vi "BlockAngle.vi"(7 "target":dbl[](array[numeric]), 8 "error in (no error)":errorcluster, 9 "Game ref":refnum<class "Game.lvclass">, 10 "Robot in":refnum<class "Robot.lvclass">, 11 "DefendAreaTactic in":refnum<class "DefendAreaTactic.lvclass">) -> (0 "error out":errorcluster, 2 "Robot out":refnum<class "Robot.lvclass">, 3 "DefendAreaTactic out":refnum<class "DefendAreaTactic.lvclass">)   [LabVIEW 2024, in "DefendAreaTactic.lvclass"]
uses:
  DefendAreaTactic.lvclass
  Game_class/Game.lvclass
  Robot_class/Robot.lvclass
  C:/Users/as119/OneDrive/Documentos/roboIME/SSL_AI/Object_class/Object.lvclass
  WallPositions.ctl
  Game_class/Game.lvclass/Game.ctl
  Team_class/Team.lvclass/Team.ctl
  Robot_class/Robot.lvclass/Robot.ctl
  Object_class/Object.lvclass/Object.ctl
  Field_class/Field.lvclass/Field.ctl
  Robot_class/Read id.vi
  Object_class/Read position(x,y).vi
  Object_class/Read y.vi
  Robot_class/Read v_norm.vi
  Robot_class/Read orientation.vi
  Game_class/Read FieldRef.vi
  Game_class/Read DefensiveTeam.vi
  Game_class/Read NewParameters.vi
  Team_class/Read RobotRef.vi
  Robot_class/Read dest_x.vi
  Robot_class/Read dest_y.vi
  Field_class/Read ourGoalPosition.vi
  Robot_class/Write dest_orientation.vi
  Robot_class/Write dest_x.vi
  Robot_class/Write dest_y.vi
  Robot_class/Write kick_x.vi
  Robot_class/Write kick_z.vi
  Ally_class/Ally.lvclass
  C:/Users/as119/OneDrive/Documentos/roboIME/SSL_AI/Team_class/Team.lvclass
  Field_class/Field.lvclass
  <vilib>/Analysis/NI_AALPro.lvlib
  Utilities_class/Utilities.lvclass
  <vilib>/Analysis/coordinate.llb/2D Cartesian Coordinate Rotation (Scalar).vi
  Ball_class/Ball.lvclass
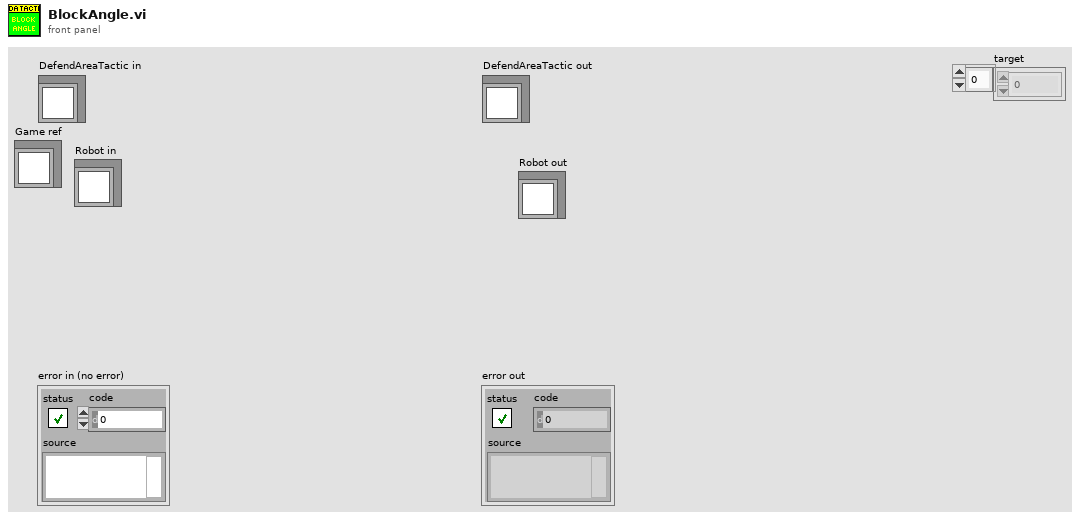
[diagram p1: front panel]
types:
  T1 = typedef "WallPositions.ctl" = enum16{"LeftWall", "LeftCorner", "FrontWall", "RightCorner", "RightWall"}
  T2 = typedef "NewParameters.ctl" = cluster{"PenaltyDistance":dbl, "DistanceAttackerToBackBall":dbl, "Division":enum16{"Div B", "Div A"}, "DistanceToAvoidyEnemyRobot":dbl, "BallPlacementDistance":dbl, "DisatanceBehindBallToStealBall":dbl, "MaxDistanceToPositionKickoff":dbl, "BlockEnemyTarget":bool, "MaxStopVAng":dbl, "DistanceMarkerToEnemy":dbl, "IgnoreDribblerContact":bool, "DistanceToBeginEnemyPosession":dbl, "GoToBallWhenEnemyNotMoving":bool, "EnemyDistanceToReduceVelocity":dbl, "TurnOnEnemyDistanceToReduceVelocity":bool, "EnemyDistanceToShootOutBall":dbl, "DefenseKickBall":bool, "MoreKickToGoal? (0-0.3)":dbl, "ChipKickInEnemyField":bool, "ShootOutRobotId":dbl, "FieldLenghtDenominatorInShootOut":dbl, "AdjustPositionInBallPlacement":bool, "PowerGodPass":dbl, "VelocityAbortEnemyPos":dbl, "MaxDistToBeginPass":dbl, "MinDistToBeginPass":dbl, "VelocityInDirects":dbl, "BadDribblerIDs":i32[], "NewKickToDistanceAroundBall":dbl, "PowerAvoidColisionMarker":dbl, "DistanceToAvoidColisionMarker":dbl, "AvoidBallKick":dbl, "DistanceTryKick":dbl, "SuicideKickDIstance":dbl, "AdjustFirstKickDistance":dbl, "AvoidAimLessKick":dbl, "DistanceToAvoidyEnemyShootRobot ":dbl, "NumberOfMarkers":dbl, "PotField":bool, "PIDLateral":bool, "MinDistanceFirstKickX":dbl, "MinDistanceFirstKickY":dbl, "FractionOfDistToTouchGround\nAfterChipKick":dbl, "FractionOfKickxWhen\nComposedWithKickz":dbl, "Style":T3, "MoveInTurnState":bool, "DistFromEnemyToConsider\nMoveInTurnState":dbl, "CascadePID":bool, "TurnAroundParameters":cluster{"Radius":dbl, "Multiplier":dbl, "ChordAngle":dbl}, "SafeDriveVel":dbl, "DistanceToGoToBackBall":dbl, "minDistanceToNotFinish\nEnemyPossession":dbl, "OneTouchShot":cluster{"angleFactor":dbl, "maxAngle":dbl, "Attack":bool, "Defense":bool}, "OpenAngleToGoal":cluster{"minAngle":dbl, "maxAngle":dbl, "minEvaluation":dbl}, "ShotInterception":cluster{"shotSpeed":dbl, "minEnemySpeed":dbl, "maxEnemySpeed":dbl, "minEvaluation":dbl}, "AllyTeamArray":T4[], "maxDefendersNumber":i32, "Zone":cluster{"GuardPositionArray":dbl[][], "ZoneMidField":dbl[], "CenterForwardWidth":dbl}, "MinEvaluationToShoot":dbl, "PassInterception":cluster{"maxPassSpeed":dbl, "minPassSpeed":dbl, "minEnemySpeed":dbl, "chipPassDistance":dbl, "chipPassEvaluation":dbl, "minEvaluation":dbl, "maxEnemySpeed":dbl}, "PassDistance":cluster{"maxDistance":dbl, "minDistance":dbl}, "receiverSpeed":dbl, "maxBallSpeed":dbl, "slackTime":dbl, "Turning radius":dbl, "Turning v_ang":dbl, "AlignError":cluster{"Distance":dbl, "Orientation":dbl, "V_norm(m/s)":dbl, "V_ang (rad/s)":dbl}, "RobotRadius":dbl, "KickerDistance":dbl, "keeper angle  to cover goalpost":dbl, "a_slide":dbl, "a_roll":dbl, "k_switch":dbl}
  T3 = typedef "Style.ctl" = enum16{"Insanity", "Offensive", "Defensive"}
  T4 = typedef "AllyTeam.ctl" = enum16{"Keeper", "Defender", "Attacker"}
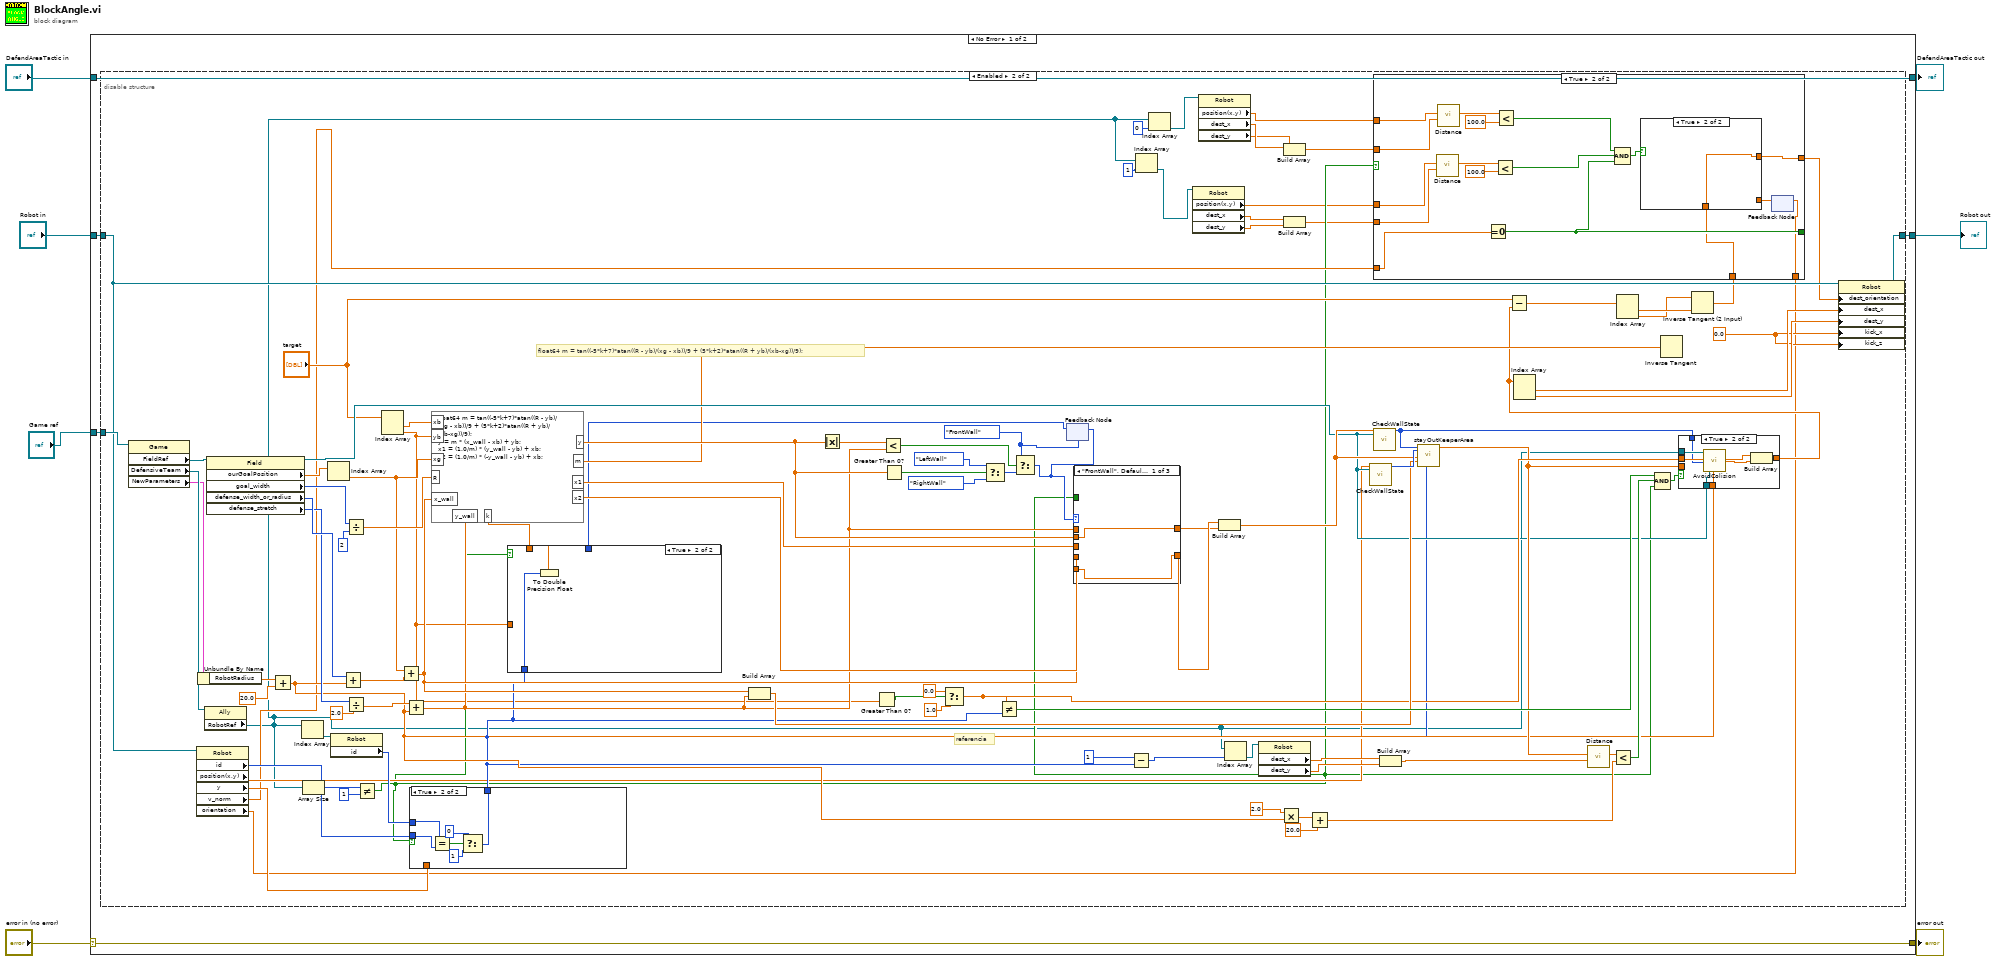
[diagram p0: block diagram]
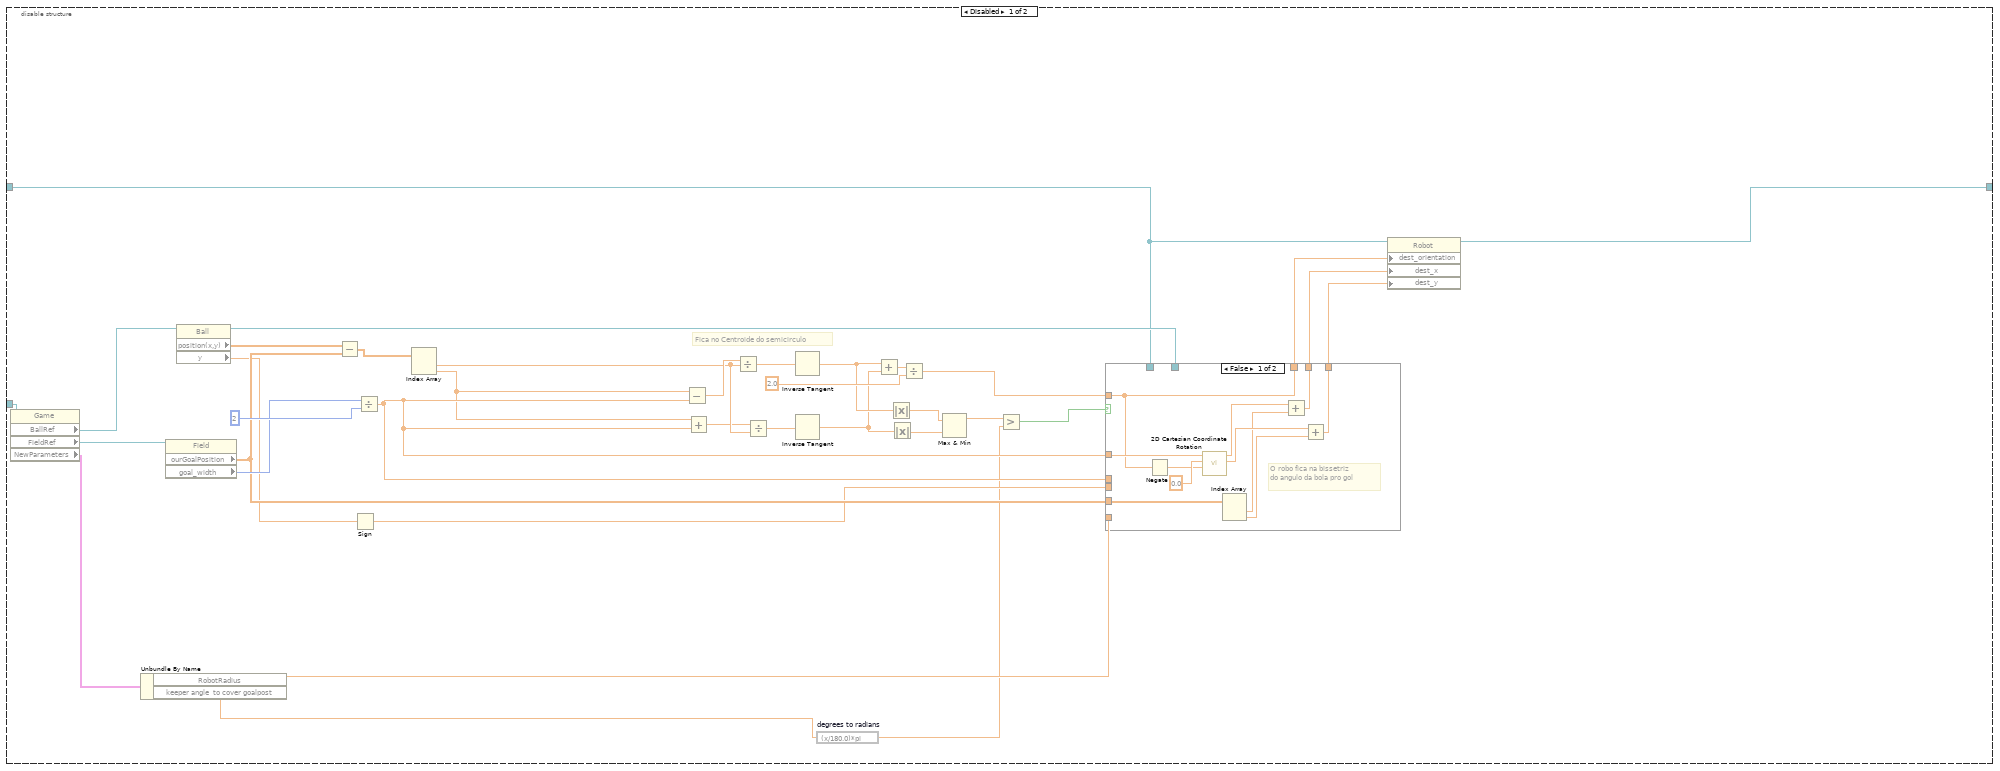
[diagram p2: hidden frame]
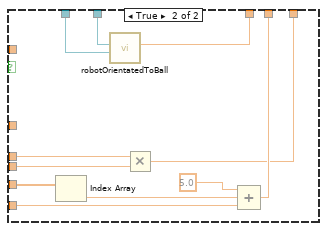
[diagram p3: hidden frame]
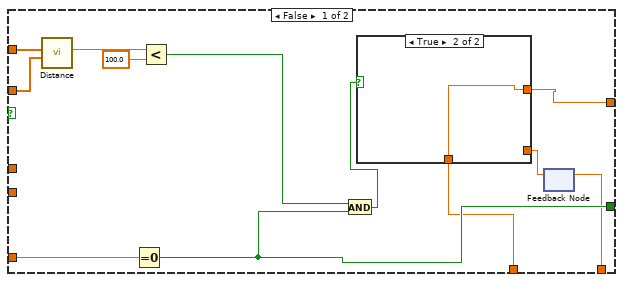
[diagram p4: hidden frame]
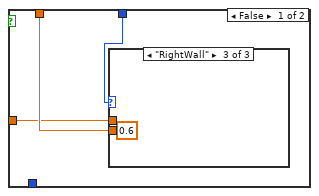
[diagram p7: hidden frame]
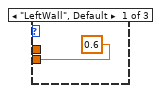
[diagram p8: hidden frame]
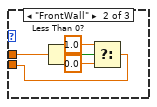
[diagram p9: hidden frame]
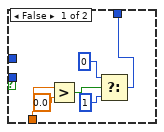
[diagram p10: hidden frame]
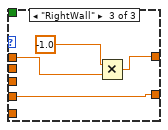
[diagram p13: hidden frame]
diagram:
  n1 = case shown="No Error" "error in (no error)" {
    selector: "error in (no error)" -> [w11 w244]
    tunnel: [w11 w244] -> w6
    tunnel: [w12 w243] -> w4
    tunnel: "DefendAreaTactic in" -> [w12 w243]
    tunnel: "Game ref" -> [w10 _]
    tunnel: "Robot in" -> [w8 w242]
    tunnel: [w9 w242] -> w1
    frame No Error {
      n2 = disable-structure shown="Enabled" {
        disable-tunnel: w10 -> [w23 w167]
        disable-tunnel: [w22 w157] -> w9
        disable-tunnel: w8 -> [w21 w155]
        frame Disabled {
          # "Fica no Centroide do semicirculo"
          n3 = property class="Game"(reference=w23) -> ("BallRef"=w48:refnum<class "Ball.lvclass">, "FieldRef"=w47:refnum<class "Field.lvclass">, "NewParameters"=w29:T2)  [unwired: 1 in, 2 out]
          n4 = Unbundle By Name(w29) -> ("RobotRadius"=w28:dbl, "keeper angle  to cover goalpost"=w13:dbl)
          n5 = property class="Field"(reference=w47) -> ("ourGoalPosition"=w35:dbl[], "goal_width"=w36:i32)  [unwired: 1 in, 2 out]
          n6 = property class="Ball"(reference=w48) -> (reference out=w30:refnum<class "Ball.lvclass">, "position(x,y)"=w46:dbl[], "y"=w25:dbl)  [unwired: 1 in, 1 out]
          n7 = Subtract(x=w46, y=w35) -> (x-y=w44:dbl[])
          n8 = Sign(1:w25) -> (0:w24:dbl)
          n9 = Divide(x=w36, y=2) -> (x/y=w27:dbl)
          n10 = Index Array(array=w44) -> (element #1=w42:dbl, element #2=w26:dbl)  [unwired: 2 in]
          n11 = Subtract(x=w26, y=w27) -> (x-y=w43:dbl)
          n12 = Add(x=w26, y=w27) -> (x+y=w41:dbl)
          n13 = Divide(x=w43, y=w42) -> (x/y=w45:dbl)
          n14 = Divide(x=w41, y=w42) -> (x/y=w40:dbl)
          n15 = Inverse Tangent(1:w45) -> (0:w20:dbl)
          n16 = Inverse Tangent(1:w40) -> (0:w19:dbl)
          n17 = expression code="(x/180.0)*pi" "degrees to radians"(w13) -> (w15:dbl)
          n18 = Add(x=w20, y=w19) -> (x+y=w38:dbl)
          n19 = Absolute Value(x=w20) -> (abs(x)=w18:dbl)
          n20 = Absolute Value(x=w19) -> (abs(x)=w17:dbl)
          n21 = Divide(x=w38, y=2.0) -> (x/y=w32:dbl)
          n22 = Max & Min(x=w18, y=w17) -> (max(x,y)=w16:dbl)  [unwired: 1 out]
          n23 = Greater?(x=w16, y=w15) -> (0:w14:bool)
          n24 = case shown="False" w14 {
            tunnel: w27 -> [w58 _]
            tunnel: w35 -> [w57 w67]
            tunnel: [w51 w64] -> w34
            tunnel: [w50 w61] -> w33
            tunnel: w32 -> [w49 _]
            tunnel: [w49 w69] -> w31
            tunnel: w30 -> [_ w70]
            tunnel: w28 -> [_ w68]
            tunnel: w27 -> [_ w62]
            tunnel: w24 -> [_ w63]
            tunnel: w21 -> [_ w60]
            frame False {
              # "O robo fica na bissetriz \ndo angulo da bola pro gol"
              n25 = Negate(x=w49) -> (-x=w54:dbl)
              n26 = call-poly <vilib>:"2D Cartesian Coordinate Rotation.vi"("theta"=w54, "y"=0.0, "x"=w58) -> ("y out"=w55:dbl, "x out"=w56:dbl)  [unwired: 6 in, 1 out]
              n27 = Index Array(array=w57) -> (element #1=w53:dbl, element #2=w52:dbl)  [unwired: 2 in]
              n28 = Add(x=w56, y=w53) -> (x+y=w51:dbl)
              n29 = Add(x=w55, y=w52) -> (x+y=w50:dbl)
            }
            frame True {
              n30 = Index Array(array=w67) -> (element=w66:dbl)  [unwired: 1 in]
              n31 = call "robotOrientatedToBall.vi"("Robot"=w60, "BallRef"=w70) -> ("Orientation"=w69:dbl)  [unwired: 7 in, 2 out]
              n32 = Multiply(x=w62, y=w63) -> (x*y=w61:dbl)
              n33 = Compound Arithmetic op=ADD(5.0 ("value"), w66, w68) -> (w64:dbl)
            }
          }
          n34 = property class="Robot"(reference=w21, "dest_orientation"=w31, "dest_x"=w34, "dest_y"=w33) -> (reference out=w22:refnum<class "Robot.lvclass">)  [unwired: 1 in, 1 out]
        }
        frame Enabled {
          w89 = 0.0 ("kick_x")
          w94 = WallPositions."FrontWall"
          # "float64 m = tan((-5*k+7)*atan((R - yb)/(xg - xb))/9 + (5*k+2)*atan((R + yb)/(xb-xg))/9);"
          # "referencia"
          n35 = property class="Game"(reference=w167) -> ("FieldRef"=w166:refnum<class "Field.lvclass">, "DefensiveTeam"=w156:refnum<class "Ally.lvclass">, "NewParameters"=w135:T2)  [unwired: 1 in, 2 out]
          n36 = property class="Robot"(reference=w155) -> ("id"=w152:i32, "position(x,y)"=w91:dbl[], "y"=w121:dbl, "v_norm"=w88:dbl, "orientation"=w71:dbl)  [unwired: 1 in, 2 out]
          n37 = Unbundle By Name(w135) -> ("RobotRadius"=w107:dbl)
          n38 = property class="Ally"(reference=w156) -> ("RobotRef"=w85:refnum<class "Robot.lvclass">[])  [unwired: 1 in, 2 out]
          n39 = property class="Field"(reference=w166) -> (reference out=w109:refnum<class "Field.lvclass">, "ourGoalPosition"=w164:dbl[], "goal_width"=w163:i32, "defense_width_or_radius"=w151:i32, "defense_stretch"=w149:i32)  [unwired: 1 in, 1 out]
          n40 = Add(x=w107, y=20.0) -> (x+y=w106:dbl)
          n41 = Index Array(array=w85) -> (element=w154:refnum<class "Robot.lvclass">)  [unwired: 1 in]
          n42 = Array Size(array=w85) -> (size(s)=w123:i32)
          n43 = Index Array(array=w164) -> (element=w147:dbl)  [unwired: 1 in]
          n44 = property class="Robot"(reference=w154) -> ("id"=w153:i32)  [unwired: 1 in, 2 out]
          n45 = Add(x=w151, y=w106) -> (x+y=w146:dbl)
          n46 = Divide(x=w163, y=2) -> (x/y=w161:dbl)
          n47 = Divide(x=w149, y=2.0) -> (x/y=w120:dbl)
          n48 = Not Equal?(x=w123, y=1) -> (x != y?=w87:bool)
          n49 = Index Array(array="target") -> (element #1=w165:dbl, element #2=w92:dbl)  [unwired: 2 in]
          n50 = Add(x=w147, y=w146) -> (x+y=w128:dbl)
          n51 = Add(x=w120, y=w106) -> (x+y=w111:dbl)
          n52 = case shown="True" w87 {
            tunnel: w153 -> [_ w224]
            tunnel: w152 -> [_ w222]
            tunnel: [w214 w219] -> w98
            tunnel: w121 -> [w218 _]
            frame False {
              n53 = Greater?(x=w218, y=0.0) -> (0:w216:bool)
              n54 = Select(t=0 ("y"), s=w216, f=1 ("y")) -> (s? t:f=w214:i32)
            }
            frame True {
              n55 = Equal?(x=w224, y=w222) -> (x = y?=w223:bool)
              n56 = Select(t=0, s=w223, f=1) -> (s? t:f=w219:i32)
            }
          }
          n57 = Build Array(w128, w111) -> (w127:dbl[])
          n58 = Greater Than 0?(x=w92) -> (x > 0?=w103:bool)
          n59 = Select(t=0.0, s=w103, f=1.0) -> (s? t:f=w126:dbl)
          n60 = Not Equal?(x=w126, y=w98) -> (x != y?=w136:bool)
          n61 = feedback #1(w94) -> (w93:T1)
          n62 = case shown="True" w87 {
            tunnel: w98 -> [_ w212]
            tunnel: [w202 w211] -> w97
            tunnel: w93 -> [w203 _]
            tunnel: w92 -> [w201 _]
            frame False {
              n63 = case shown="\"RightWall\"" w203 {
                tunnel: [0.6 w205 0.6] -> w202
                tunnel: w201 -> [_ w209 _]
                frame "LeftWall", Default {
                }
                frame "FrontWall" {
                  n64 = Less Than 0?(x=w209) -> (x < 0?=w208:bool)
                  n65 = Select(t=1.0, s=w208, f=0.0) -> (s? t:f=w205:dbl)
                }
                frame "RightWall" {
                }
              }
            }
            frame True {
              n66 = To Double Precision Float(number=w212) -> (double precision float=w211:dbl)
            }
          }
          n67 = formula code="float64 m = tan((-5*k+7)*atan((R - yb)/(xg - xb))/9 + (5*k+2)*atan((R + yb)/(xb-xg))/9);\ny = m * (x_wall - xb) + yb;\nx1 = (1.0/m) * (y_wall - yb) + xb;\nx2 = (1.0/m) * (-y_wall - yb) + xb;"("xb"=w165, "yb"=w92, "xg"=w147, "R"=w161, "k"=w97, "x_wall"=w128, "y_wall"=w111) -> ("y"=w142:dbl, "x1"=w141:dbl, "x2"=w140:dbl, "m"=w96:dbl)
          n68 = Absolute Value(x=w142) -> (abs(x)=w148:dbl)
          n69 = Less?(x=w148, y=w111) -> (x < y?=w145:bool)
          n70 = Greater Than 0?(x=w142) -> (x > 0?=w137:bool)
          n71 = Select(t=WallPositions."LeftWall", s=w137, f=WallPositions."RightWall") -> (s? t:f=w143:T1)
          n72 = Select(t=w94, s=w145, f=w143) -> (s? t:f=w95:T1)
          n73 = feedback-in #1(w95) -> ()
          n74 = case shown="\"FrontWall\", Default" w95 {
            tunnel: w142 -> [w234 _ _]
            tunnel: w141 -> [_ w236 _]
            tunnel: w140 -> [_ _ w238]
            tunnel: w111 -> [_ w237 w240]
            tunnel: w128 -> [w235 _ _]
            tunnel: [w234 w237 w239] -> w133
            tunnel: [w235 w236 w238] -> w134
            tunnel: w87 -> [_ _ _]
            frame "FrontWall", Default {
            }
            frame "LeftWall" {
            }
            frame "RightWall" {
              n75 = Multiply(x=-1.0, y=w240) -> (x*y=w239:dbl)
            }
          }
          n76 = Subtract(x=1, y=w98) -> (x-y=w105:i32)
          n77 = Index Array(array=w85, index=1) -> (element=w83:refnum<class "Robot.lvclass">)
          n78 = Index Array(array=w85, index=0) -> (element=w82:refnum<class "Robot.lvclass">)
          n79 = property class="Robot"(reference=w83) -> ("position(x,y)"=w77:dbl[], "dest_x"=w80:dbl, "dest_y"=w79:dbl)  [unwired: 1 in, 2 out]
          n80 = property class="Robot"(reference=w82) -> ("position(x,y)"=w81:dbl[], "dest_x"=w76:dbl, "dest_y"=w75:dbl)  [unwired: 1 in, 2 out]
          n81 = Build Array(w134, w133) -> (w110:dbl[])
          n82 = Index Array(array=w85, index=w105) -> (element=w118:refnum<class "Robot.lvclass">)
          n83 = property class="Robot"(reference=w118) -> ("dest_x"=w102:dbl, "dest_y"=w101:dbl)  [unwired: 1 in, 2 out]
          n84 = Multiply(x=2.0, y=w106) -> (x*y=w115:dbl)
          n85 = Build Array(w76, w75) -> (w74:dbl[])
          n86 = Build Array(w80, w79) -> (w78:dbl[])
          n87 = Add(x=w115, y=20.0) -> (x+y=w113:dbl)
          n88 = call "CheckWallState.vi"("Position"=w91, "Field"=w109) -> ("WallState"=w131:T1)  [unwired: 16 in, 1 out]
          n89 = call "CheckWallState.vi"("Position"=w110, "Field"=w109) -> ("WallState"=w125:T1)  [unwired: 16 in, 1 out]
          n90 = Build Array(w102, w101) -> (w100:dbl[])
          n91 = call "stayOutKeeperArea.vi"("DesireState"=w125, "CurrentState"=w131, "Dest"=w110, "LeftCornerPosition"=w127, "reference"=w98) -> ("CorrectDest"=w119:dbl[])  [unwired: 13 in, 1 out]
          n92 = call "Distance.vi"("P1"=w100, "P2"=w119) -> ("Distance"=w117:dbl)  [unwired: 7 in, 2 out]
          n93 = Less?(x=w117, y=w113) -> (x < y?=w112:bool)
          n94 = Compound Arithmetic op=AND(w136, w112, w87) -> (w124:bool)
          n95 = Inverse Tangent(1:w96) -> ()  [unwired: 1 out]
          n96 = case shown="True" w124 {
            tunnel: w85 -> [_ w233]
            tunnel: w126 -> [_ w232]
            tunnel: w125 -> [_ w231]
            tunnel: w106 -> [_ w230]
            tunnel: [w225 w227] -> w90
            tunnel: w119 -> [w225 _]
            tunnel: w109 -> [_ w226]
            frame False {
            }
            frame True {
              n97 = call "AvoidColision.vi"("RobotRef"=w233, "referencia"=w232, "positionOnWall"=w231, "Field"=w226, "robot Radius"=w230) -> ("dest_x"=w229:dbl, "dest_y"=w228:dbl)  [unwired: 12 in, 1 out]
              n98 = Build Array(w229, w228) -> (w227:dbl[])
            }
          }
          n99 = Subtract(x="target", y=w90) -> (x-y=w160:dbl[])
          n100 = Index Array(array=w90) -> (element #1=w130:dbl, element #2=w129:dbl)  [unwired: 2 in]
          n101 = Index Array(array=w160) -> (element #1=w159:dbl, element #2=w158:dbl)  [unwired: 2 in]
          n102 = Inverse Tangent (2 Input)(1:w159, 2:w158) -> (0:w72:dbl)
          n103 = case shown="True" w87 {
            tunnel: w88 -> [w177 w196]
            tunnel: w81 -> [w175 w191]
            tunnel: w78 -> [_ w193]
            tunnel: w77 -> [_ w192]
            tunnel: w74 -> [w174 w188]
            tunnel: [w173 w187] -> _
            tunnel: [w169 w184] -> w73
            tunnel: w72 -> [w170 w185]
            tunnel: w71 -> [w168 w182]
            frame False {
              n104 = call "Distance.vi"("P1"=w174, "P2"=w175) -> ("Distance"=w179:dbl)  [unwired: 7 in, 2 out]
              n105 = Equal To 0?(x=w177) -> (x = 0?=w173:bool)
              n106 = Less?(x=w179, y=100.0) -> (x < y?=w176:bool)
              n107 = And(x=w176, y=w173) -> (x .and. y?=w171:bool)
              n108 = feedback #2() -> (w172:dbl)  [unwired: 1 in]
              n109 = case shown="True" w171 {
                tunnel: [w180 w181] -> w169
                tunnel: w170 -> [_ w181]
                tunnel: w172 -> [w180 _]
                frame False {
                }
                frame True {
                }
              }
              n110 = feedback-in #2(w168) -> ()
            }
            frame True {
              n111 = call "Distance.vi"("P1"=w193, "P2"=w192) -> ("Distance"=w198:dbl)  [unwired: 7 in, 2 out]
              n112 = call "Distance.vi"("P1"=w188, "P2"=w191) -> ("Distance"=w194:dbl)  [unwired: 7 in, 2 out]
              n113 = Equal To 0?(x=w196) -> (x = 0?=w187:bool)
              n114 = Less?(x=w198, y=100.0) -> (x < y?=w190:bool)
              n115 = Less?(x=w194, y=100.0) -> (x < y?=w189:bool)
              n116 = Compound Arithmetic op=AND(w189, w190, w187) -> (w186:bool)
              n117 = feedback-in #3(w182) -> ()
              n118 = feedback #3() -> (w183:dbl)  [unwired: 1 in]
              n119 = case shown="True" w186 {
                tunnel: [w199 w200] -> w184
                tunnel: w185 -> [_ w200]
                tunnel: w183 -> [w199 _]
                frame False {
                }
                frame True {
                }
              }
            }
          }
          n120 = property class="Robot"(reference=w155, "dest_orientation"=w73, "dest_x"=w130, "dest_y"=w129, "kick_x"=w89, "kick_z"=w89) -> (reference out=w157:refnum<class "Robot.lvclass">)  [unwired: 1 in, 1 out]
        }
      }
    }
    frame Error {
    }
  }
  "error out" <- w6
  "DefendAreaTactic out" <- w4
  "Robot out" <- w1
